vi "PFI-28000-Base_Write Command.vi"(0 "PFI-28000-Base in":refnum<class "PFI-28000-Base.lvclass">, 5 "Command":string, 11 "error in (no error)":errorcluster) -> (4 "PFI-28000-Base out":refnum<class "PFI-28000-Base.lvclass">, 15 "error out":errorcluster)   [LabVIEW 2017, in "PFI-28000-Base.lvclass"]
uses:
  PFI-28000-Base.lvclass
  Utilities/PFI-28000-Utils.lvlib
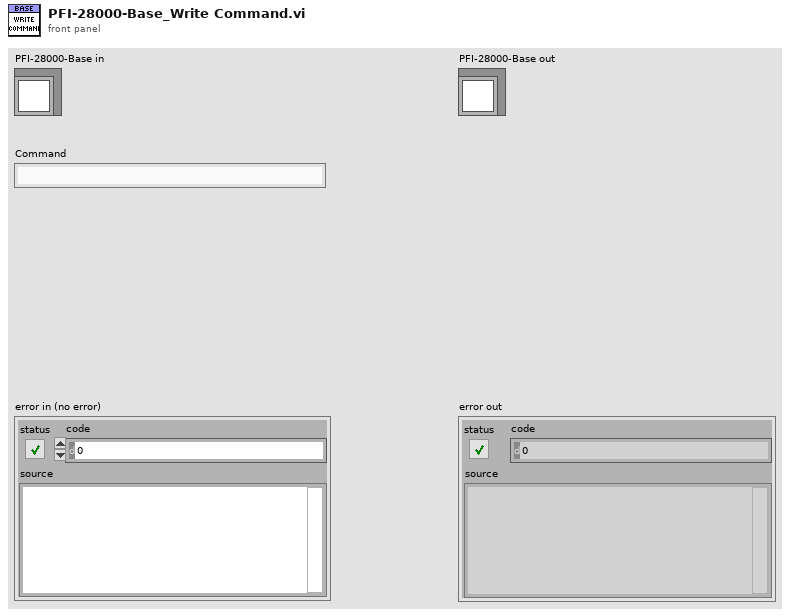
[diagram p1: front panel]
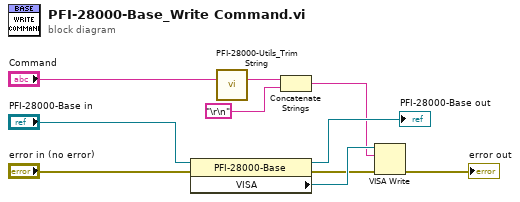
[diagram p0: block diagram]
diagram:
  n1 = property class="PFI-28000-Base"(reference="PFI-28000-Base in", error in="error in (no error)") -> (reference out=→"PFI-28000-Base out":refnum<class "PFI-28000-Base.lvclass">, error out=w9:errorcluster, "VISA"=w10:refnum<visa-resource-name>)
  n2 = call "PFI-28000-Utils_Trim String.vi"("String"="Command") -> ("Trimmed String"=w3:string)  [unwired: 14 in]
  n3 = Concatenate Strings(w3, "\r\n") -> (w2:string)
  n4 = VISA Write(VISA resource name=w10, write buffer=w2, error in (no error)=w9) -> (error out=→"error out":errorcluster)  [unwired: 2 out]
